vi "check_sweepcount.vi"(0 "rangenumber":i32, 1 "sopcount":i32, 2 "Meas_rang":i32[](array[numeric]), 3 "chk2scan":bool) -> (8 "sweepcount":i32)   [LabVIEW 2017]
doc: "Return Sweep count for range and SOP status"
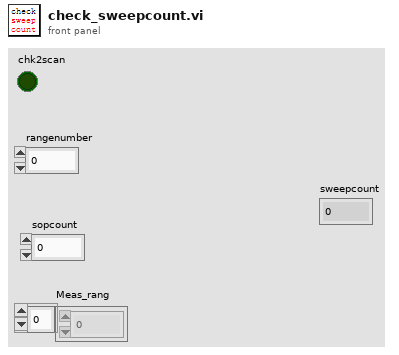
[diagram p1: front panel]
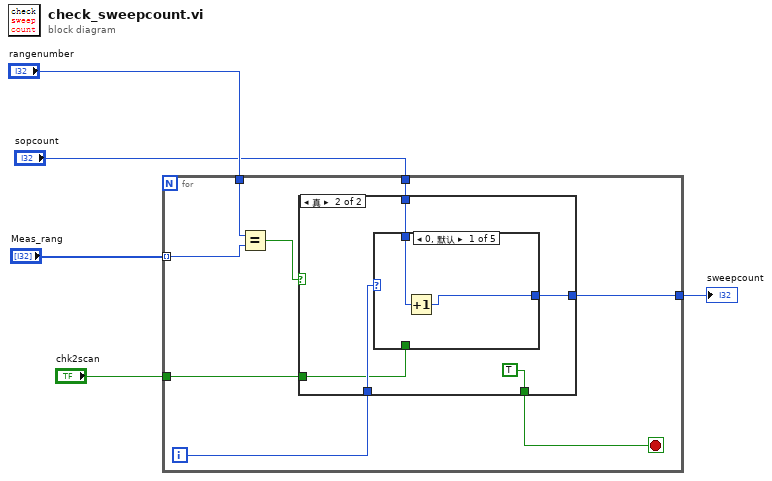
[diagram p0: block diagram]
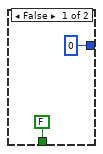
[diagram p2: hidden frame]
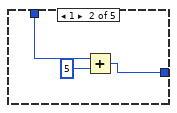
[diagram p3: hidden frame]
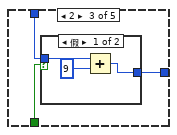
[diagram p4: hidden frame]
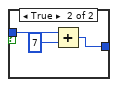
[diagram p5: hidden frame]
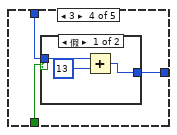
[diagram p6: hidden frame]
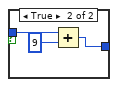
[diagram p7: hidden frame]
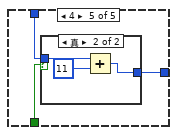
[diagram p8: hidden frame]
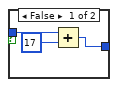
[diagram p9: hidden frame]
diagram:
  n1 = for {
    tunnel: "Meas_rang" -> [w12] mode=indexing
    tunnel: "rangenumber" -> [w13]
    tunnel: "sopcount" -> [w9]
    tunnel: [w8] -> w2
    tunnel: "chk2scan" -> [w7]
    i -> [w10]
    stop <- w6 stop-if-true
    n2 = Equal?(x=w13, y=w12) -> (x = y?=w11:bool)
    n3 = case shown="真" w11 {
      tunnel: w10 -> [_ w20]
      tunnel: w9 -> [_ w19]
      tunnel: [0 w18] -> w8
      tunnel: w7 -> [_ w17]
      tunnel: [FALSE TRUE] -> w6
      frame False {
      }
      frame True {
        n4 = case shown="0, 默认" w20 {
          tunnel: w19 -> [w22 w25 w28 w37 w46]
          tunnel: [w21 w23 w26 w35 w44] -> w18
          tunnel: w17 -> [_ _ w27 w36 w45]
          frame 0, Default {
            n5 = Increment(x=w22) -> (x+1=w21:i32)
          }
          frame 1 {
            n6 = Add(x=w25, y=5) -> (x+y=w23:i32)
          }
          frame 2 {
            n7 = case shown="假" w27 {
              tunnel: w28 -> [w31 w34]
              tunnel: [w29 w32] -> w26
              frame False {
                n8 = Add(x=w31, y=9) -> (x+y=w29:i32)
              }
              frame True {
                n9 = Add(x=w34, y=7) -> (x+y=w32:i32)
              }
            }
          }
          frame 3 {
            n10 = case shown="假" w36 {
              tunnel: w37 -> [w40 w43]
              tunnel: [w38 w41] -> w35
              frame False {
                n11 = Add(x=w40, y=13) -> (x+y=w38:i32)
              }
              frame True {
                n12 = Add(x=w43, y=9) -> (x+y=w41:i32)
              }
            }
          }
          frame 4 {
            n13 = case shown="真" w45 {
              tunnel: w46 -> [w49 w52]
              tunnel: [w47 w50] -> w44
              frame False {
                n14 = Add(x=w49, y=17) -> (x+y=w47:i32)
              }
              frame True {
                n15 = Add(x=w52, y=11) -> (x+y=w50:i32)
              }
            }
          }
        }
      }
    }
  }
  "sweepcount" <- w2
